vi "Initialize Incoming.vi"(8 "error in (no error)":errorcluster, 11 "OnCompile Variables":T15={"XNET Settings"={"Database"="", "Cluster"="", "Port"="", "Baud rate [Bd]"=500000, "Termination"=1, "CAN I/O Mode"=0, "FD Baud rate [Bd]"=500000, "Priority"=100, "Use Legacy"=FALSE}, "Frames"=[], "986x Support"={"Enable"=FALSE, "RIO Device"="", "Bitfile"=path ""}, "Incoming Frames"=[], "Incoming Signal Info"={"Signal Settings Out"=[], "Signal.PrevData"=[], "Signal Names"=[]}} {"Incoming Signal Info"."Signal Settings Out"."Protection Configuration"."CRC Channels"."Data Type" items=["Signed", "Unsigned", "IEEE Float"]; "Incoming Frames"."Protection Configurations"."CRC Channels"."Data Type" items=["Signed", "Unsigned", "IEEE Float"]; "XNET Settings"."CAN I/O Mode" items=["CAN 2.0", "CAN FD", "CAN FD+BRS"]; "XNET Settings"."Termination" items=["Off", "On"]; "Frames"."Protection Configurations"."CRC Channels"."Data Type" items=["Signed", "Unsigned", "IEEE Float"]}) -> (0 "error out":errorcluster, 1 "RT Incoming Signal Info":T7 {"Signal Settings Out"."Protection Configuration"."CRC Channels"."Data Type" items=["Signed", "Unsigned", "IEEE Float"]}, 2 "Incoming CAN Session":refnum<k21>, 3 "Signal Values":dbl[](array[numeric]))   [LabVIEW 2015, in "Protection and Counter Addon Engine.lvlib"]
uses:
  Protection and Counter Addon Engine.lvlib
  Shared/Types/Exported.OnCompile.ctl
  Shared/Types/XNET Settings.ctl
  SubModules/Frame Protection Support/Source/Shared/Types/Exported Frame Settings.ctl
  SubModules/Frame Protection Support/Source/Shared/Types/Exported Frame Type.ctl
  SubModules/Frame Protection Support/Source/Shared/Types/Exported Protection Settings.ctl
  SubModules/Frame Protection Support/Source/Shared/Types/Protection Type.ctl
  SubModules/Frame Protection Support/Source/Shared/Types/XNET Signal Configuration.ctl
  SubModules/Frame Protection Support/Source/Shared/Types/Exported Counter Settings.ctl
  SubModules/Frame Protection Support/Source/Shared/Types/Exported Event Trigger Type.ctl
  Shared/Types/986x.ctl
  SubModules/Frame Protection Support/Source/Shared/Types/Incoming Signal Info.ctl
  SubModules/Frame Protection Support/Source/Shared/Types/Exported Signal Settings.ctl
  Types/RT Async Engine Variables.ctl
  SubModules/Frame Protection Support/Source/Engine/Types/RT Frame Settings.ctl
  SubModules/Frame Protection Support/Source/Engine/Types/RT Protection Configuration.ctl
  SubModules/Frame Protection Support/Source/Shared/Types/RT_Incoming_Signal_Info.ctl
  SubModules/Frame Protection Support/Source/Shared/Types/RT Exported Signal Settings.ctl
  <vilib>/xnet/xnet.llb/XNET Create Session (Signal Input XY).vi
  SubModules/Frame Protection Support/Source/Shared/Protection and Counter Support Shared.lvlib
  SubModules/Frame Protection Support/Source/Engine/Protection and Counter Support Engine.lvlib
  <resource>/objmgr/xnet.rc
  Shared/Protection and Counter Addon Shared.lvlib
panel:
  out "Incoming Signal Info 2":T1 {"Signal Settings Out"."Protection Configuration"."CRC Channels"."Data Type" items=["Signed", "Unsigned", "IEEE Float"]}
  out "RT Configuration":T10={"Priority"=100, "CAN Session"="", "Frame Count"=0, "Frames"=[], "FPGA Session"=0, "Incoming Frame Session"="", "Incoming Session Invalid"=FALSE, "Incoming Frames"=[], "Signal Values"=[], "Incoming Signal Info"={"Signal.PrevData"=[], "Signal Names"=[], "Signal Settings Out"=[]}} {"Incoming Signal Info"."Signal Settings Out"."Protection Configuration"."CRC Channels"."Data Type" items=["Signed", "Unsigned", "IEEE Float"]; "Incoming Frames"."Protection Configurations"."CRC Channels"."Data Type" items=["Signed", "Unsigned", "IEEE Float"]; "Frames"."Protection Configurations"."CRC Channels"."Data Type" items=["Signed", "Unsigned", "IEEE Float"]}
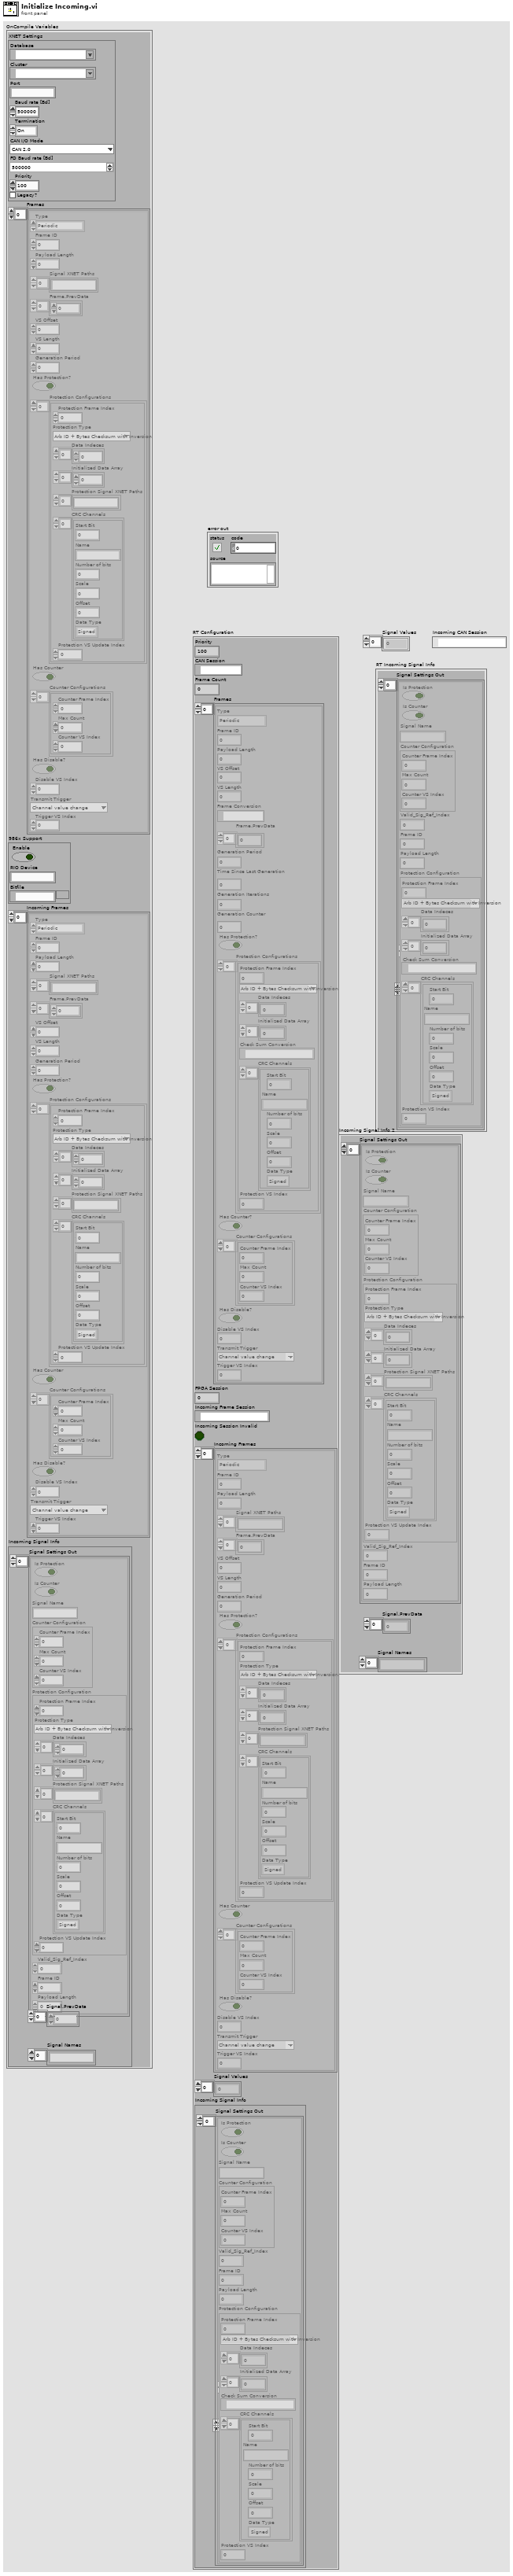
[diagram p1: front panel]
types:
  T1 = typedef "Protection and Counter Support Shared.lvlib/Incoming Signal Info.ctl" = cluster{"Signal Settings Out":T2[], "Signal.PrevData":dbl[], "Signal Names":string[]}
  T2 = typedef "Protection and Counter Support Shared.lvlib/Exported Signal Settings.ctl" = cluster{"Is Protection":bool, "Is Counter":bool, "Signal Name":string, "Counter Configuration":T3, "Protection Configuration":T4, "Valid_Sig_Ref_Index":i32, "Frame ID":u32, "Payload Length":u32}
  T3 = typedef "Protection and Counter Support Shared.lvlib/Exported Counter Settings.ctl" = cluster{"Counter Frame Index":i32, "Max Count":dbl, "Counter VS Index":i32}
  T4 = typedef "Protection and Counter Support Shared.lvlib/Exported Protection Settings.ctl" = cluster{"Protection Frame Index":i32, "Protection Type":T5, "Data Indeces":i32[], "Initialized Data Array":dbl[], "Protection Signal XNET Paths":string[], "CRC Channels":T6[], "Protection VS Update Index":i32}
  T5 = typedef "Protection and Counter Support Shared.lvlib/Protection Type.ctl" = enum16{"Arb ID + Bytes Checksum with Inversion", "Arb ID + Bytes CRC with Inversion", "Reversed Raw Signal Checksum with Inversion"}
  T6 = typedef "Protection and Counter Support Shared.lvlib/XNET Signal Configuration.ctl" = cluster{"Start Bit":i32, "Name":string, "Number of bits":i32, "Scale":dbl, "Offset":dbl, "Data Type":u32}
  T7 = typedef "Protection and Counter Support Shared.lvlib/RT_Incoming_Signal_Info.ctl" = cluster{"Signal.PrevData":dbl[], "Signal Names":string[], "Signal Settings Out":T8[]}
  T8 = typedef "Protection and Counter Support Shared.lvlib/RT Exported Signal Settings.ctl" = cluster{"Is Protection":bool, "Is Counter":bool, "Signal Name":string, "Counter Configuration":T3, "Valid_Sig_Ref_Index":i32, "Frame ID":u32, "Payload Length":u32, "Protection Configuration":T9}
  T9 = typedef "Protection and Counter Support Engine.lvlib/RT Protection Configuration.ctl" = cluster{"Protection Frame Index":i32, "Protection Type":T5, "Data Indeces":i32[], "Initialized Data Array":dbl[], "Check Sum Conversion":refnum<k21>, "CRC Channels":T6[], "Protection VS Index":i32}
  T10 = typedef "Protection and Counter Addon Engine.lvlib/RT Async Engine Variables.ctl" = cluster{"Priority":i32, "CAN Session":refnum<k21>, "Frame Count":i32, "Frames":T11[], "FPGA Session":u32, "Incoming Frame Session":refnum<k21>, "Incoming Session Invalid":bool, "Incoming Frames":T14[], "Signal Values":dbl[], "Incoming Signal Info":T7}
  T11 = typedef "Protection and Counter Support Engine.lvlib/RT Frame Settings.ctl" = cluster{"Type":T12, "Frame ID":u32, "Payload Length":u32, "VS Offset":i32, "VS Length":i32, "Frame Conversion":refnum<k21>, "Frame.PrevData":dbl[], "Generation Period":u32, "Time Since Last Generation":u32, "Generation Iterations":u32, "Generation Counter":u32, "Has Protection?":bool, "Protection Configurations":T9[], "Has Counter?":bool, "Counter Configurations":T3[], "Has Disable?":bool, "Disable VS Index":i32, "Transmit Trigger":T13, "Trigger VS Index":i32}
  T12 = typedef "Protection and Counter Support Shared.lvlib/Exported Frame Type.ctl" = enum16{"Periodic", "Event", "Periodic/Event"}
  T13 = typedef "Protection and Counter Support Shared.lvlib/Exported Event Trigger Type.ctl" = enum16{"Channel value change", "Trigger channel (not zero)", "Channel value change or trigger channel (not zero)", "Trigger channel (any value change)", "Channel value change or trigger channel (any value change)"}
  T14 = typedef "Protection and Counter Support Shared.lvlib/Exported Frame Settings.ctl" = cluster{"Type":T12, "Frame ID":u32, "Payload Length":u32, "Signal XNET Paths":string[], "Frame.PrevData":dbl[], "VS Offset":i32, "VS Length":i32, "Generation Period":u32, "Has Protection?":bool, "Protection Configurations":T4[], "Has Counter":bool, "Counter Configurations":T3[], "Has Disable?":bool, "Disable VS Index":i32, "Transmit Trigger":T13, "Trigger VS Index":i32}
  T15 = typedef "Protection and Counter Addon Shared.lvlib/Exported.OnCompile.ctl" = cluster{"XNET Settings":T16, "Frames":T14[], "986x Support":T17, "Incoming Frames":T14[], "Incoming Signal Info":T1}
  T16 = typedef "Protection and Counter Addon Shared.lvlib/XNET Settings.ctl" = cluster{"Database":refnum<k21>, "Cluster":refnum<k21>, "Port":string, "Baud rate [Bd]":u64, "Termination":u32, "CAN I/O Mode":u32, "FD Baud rate [Bd]":u64, "Priority":i32, "Use Legacy":bool}
  T17 = typedef "Protection and Counter Addon Shared.lvlib/986x.ctl" = cluster{"Enable":bool, "RIO Device":string, "Bitfile":path}
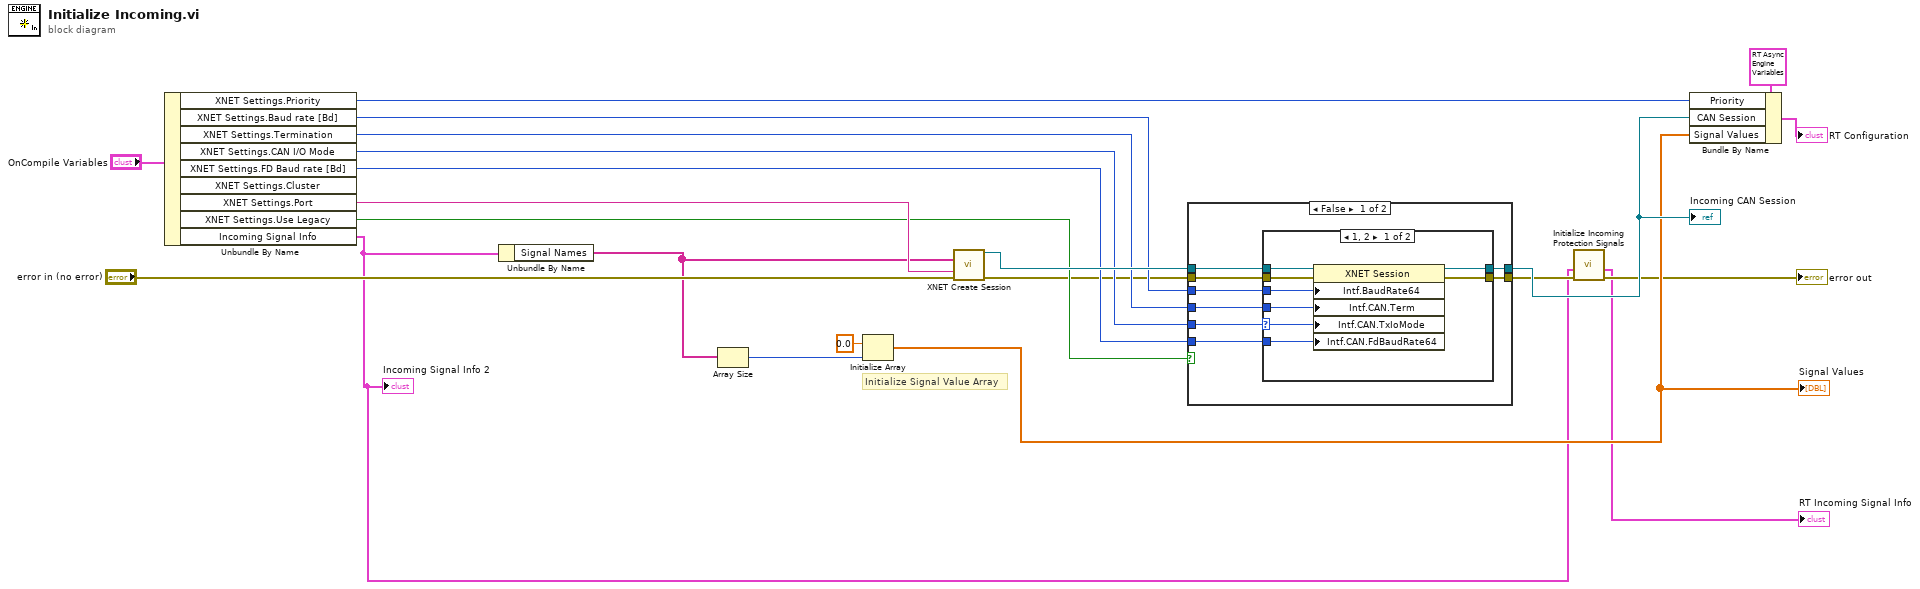
[diagram p0: block diagram]
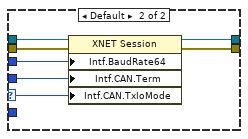
[diagram p2: hidden frame]
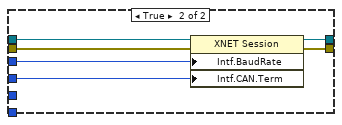
[diagram p3: hidden frame]
diagram:
  # "Initialize Signal Value Array"
  n1 = Unbundle By Name("OnCompile Variables") -> ("XNET Settings.Priority"=w13:i32, "XNET Settings.Baud rate [Bd]"=w14:u64, "XNET Settings.Termination"=w15:u32, "XNET Settings.CAN I/O Mode"=w16:u32, "XNET Settings.FD Baud rate [Bd]"=w17:u64, "XNET Settings.Port"=w18:string, "XNET Settings.Use Legacy"=w12:bool, "Incoming Signal Info"=w2:T1)  [unwired: 1 out]
  "Incoming Signal Info 2" <- w2
  n2 = Unbundle By Name(w2) -> ("Signal Names"=w5:string[])
  n3 = Array Size(array=w5) -> (size(s)=w8:i32)
  n4 = Initialize Array(0.0 ("element"), w8) -> (w6:dbl[])
  "Signal Values" <- w6
  n5 = call-poly <vilib>:"XNET Create Session.vi"("signal list"=w5, "interface"=w18, "error in (no error)"="error in (no error)") -> ("session out"=w19:refnum<k21>, "error out"=w9:errorcluster)  [unwired: 11 in]
  n6 = case shown="False" w12 {
    tunnel: w9 -> [w30 w51]
    tunnel: w19 -> [w29 w50]
    tunnel: [w28 w49] -> w4
    tunnel: w17 -> [w27 _]
    tunnel: w16 -> [w23 _]
    tunnel: w15 -> [w26 w46]
    tunnel: w14 -> [w25 w47]
    tunnel: [w24 w48] -> w11
    frame False {
      n7 = case shown="1, 2" w23 {
        selector: w23 -> [w31 w39]
        tunnel: w30 -> [w38 w45]
        tunnel: w29 -> [w37 w44]
        tunnel: [w36 w43] -> w28
        tunnel: w27 -> [w35 _]
        tunnel: w26 -> [w34 w42]
        tunnel: w25 -> [w33 w41]
        tunnel: [w32 w40] -> w24
        frame 1, 2 {
          n8 = property class="XNET Session"(reference=w37, error in=w38, "Intf.BaudRate64"=w33, "Intf.CAN.Term"=w34, "Intf.CAN.TxIoMode"=w31, "Intf.CAN.FdBaudRate64"=w35) -> (reference out=w32:refnum<k21>, error out=w36:errorcluster)
        }
        frame Default {
          n9 = property class="XNET Session"(reference=w44, error in=w45, "Intf.BaudRate64"=w41, "Intf.CAN.Term"=w42, "Intf.CAN.TxIoMode"=w39) -> (reference out=w40:refnum<k21>, error out=w43:errorcluster)
        }
      }
    }
    frame True {
      n10 = property class="XNET Session"(reference=w50, error in=w51, "Intf.BaudRate"=w47, "Intf.CAN.Term"=w46) -> (reference out=w48:refnum<k21>, error out=w49:errorcluster)
    }
  }
  "Incoming CAN Session" <- w11
  n11 = call "Initialize Incoming Protection Signals.vi"("error in (no error)"=w4, "Incoming Signal Info In"=w2) -> ("error out"=→"error out":errorcluster, "RT Incoming Signal Info"=→"RT Incoming Signal Info":T7)  [unwired: 8 in]
  n12 = Bundle By Name(cluster=T10 {"Priority"=100, "CAN Session"="", "Frame Count"=0, "Frames"=[], "FPGA Session"=0, "Incoming Frame Session"="", "Incoming Session Invalid"=FALSE, "Incoming Frames"=[], "Signal Values"=[], "Incoming Signal Info"={"Signal.PrevData"=[], "Signal Names"=[], "Signal Settings Out"=[]}} ("RT Configuration"), "Priority"=w13, "CAN Session"=w11, "Signal Values"=w6) -> (→"RT Configuration":T10)
